vi "json Insert json - string path.vi"(8 "error in (no error)":errorcluster, 9 "anything":refnum<class "JSON Document.lvclass">, 10 "path":string, 11 "JSON Document in":refnum<class "JSON Document.lvclass">) -> (0 "error out":errorcluster, 3 "JSON Document out":refnum<class "JSON Document.lvclass">)   [LabVIEW 2015, in "JSON Document.lvclass"]
uses:
  JSON Document.lvclass
  JSON Document.lvclass/JSON Document.ctl
  rapidjson wrapper/rapidjson wrapper.lvlib
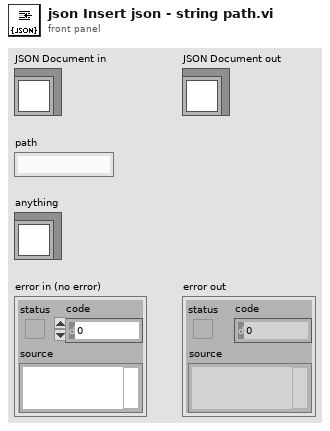
[diagram p1: front panel]
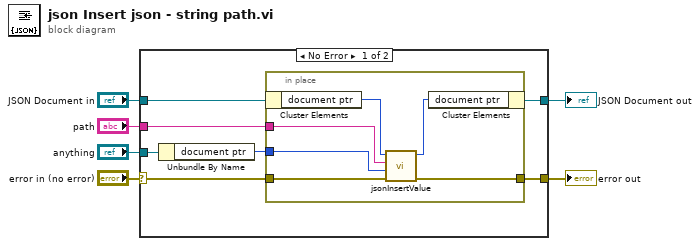
[diagram p0: block diagram]
diagram:
  n1 = case shown="No Error" "error in (no error)" {
    selector: "error in (no error)" -> [w9 w21]
    tunnel: [w10 w21] -> w5
    tunnel: [w12 w20] -> w3
    tunnel: "JSON Document in" -> [w13 w20]
    tunnel: "anything" -> [w8 _]
    tunnel: "path" -> [w11 _]
    frame No Error {
      n2 = Unbundle By Name(w8) -> ("document ptr"=w7:i64)
      n3 = in-place {
        in-place-border: w11 -> [w17]
        in-place-border: w9 -> [w16]
        in-place-border: [w15] -> w10
        in-place-border: w7 -> [w14]
        n4 = in-place-cluster #1(w13) -> ("document ptr"=w19:i64)
        n5 = call "jsonInsertValue.vi"("error in (no error)"=w16, "value"=w14, "path"=w17, "d in"=w19) -> ("error out"=w15:errorcluster, "d out"=w18:i64)  [unwired: 6 in]
        n6 = in-place-cluster #1("document ptr"=w18) -> (w12:refnum<class "JSON Document.lvclass">)
      }
    }
    frame Error {
    }
  }
  "error out" <- w5
  "JSON Document out" <- w3
